vi "GetEnumFeatureValue.vi"(9 "pFeatureName":string, 10 "handle":i64, 11 "error in (no error)":errorcluster) -> (2 "pEnumValue":u64, 3 "error out":errorcluster)   [LabVIEW 2016]
uses:
  MVSDKmd.dll
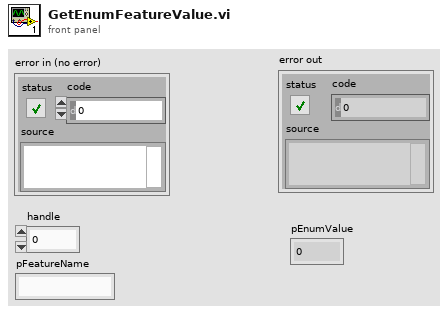
[diagram p1: front panel]
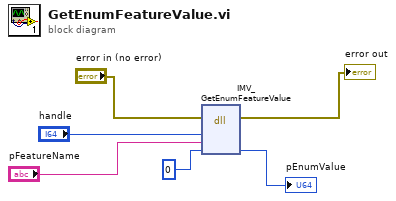
[diagram p0: block diagram]
diagram:
  n1 = dll-call lib="MVSDKmd.dll" fn="IMV_GetEnumFeatureValue"(error in="error in (no error)", "handle"="handle", "pFeatureName"="pFeatureName", "pEnumValue"=u64 0) -> (error out=→"error out":errorcluster, "pEnumValue"=→"pEnumValue":u64)  [unwired: 5 in, 1 out]
